vi "SetMotorOutFast.vi"(6 "Period (ms)":i32, 8 "error in (no error)":errorcluster, 9 "Sync Group / Parameter Slot":u8, 10 "Output":dbl, 11 "MotorControlDevRef":T1={"DeviceStatus"={"status"=FALSE, "code"=0, "source"=""}, "Type"=enum."PWM", "PWM"={"Controller"=enum."Controller 1", "PWM Channel"=enum."Invalid", "DeadBand"={"Name"="", "maxPositivePwm"=0, "minPositivePwm"=0, "centerPwm"=0, "maxNegativePwm"=0, "minNegativePwm"=0, "angularRange"=0}}, "CAN"={"Device Number"=0, "Control Mode"=enum."Percent VBus", "Semaphore"=refnum, "Max Vout"=12.0, "TalonSRX Control Mode"=enum."Percent VBus"}, "Invert"=FALSE, "TransformRef"=refnum, "InvTransformRef"=refnum}) -> (0 "error out":errorcluster, 2 "Motor Output":dbl, 3 "MotorControlDevRefOut":T1={"DeviceStatus"={"status"=FALSE, "code"=0, "source"=""}, "Type"=enum."PWM", "PWM"={"Controller"=enum."Controller 1", "PWM Channel"=enum."Invalid", "DeadBand"={"Name"="", "maxPositivePwm"=0, "minPositivePwm"=0, "centerPwm"=0, "maxNegativePwm"=0, "minNegativePwm"=0, "angularRange"=0}}, "CAN"={"Device Number"=0, "Control Mode"=enum."Percent VBus", "Semaphore"=refnum, "Max Vout"=12.0, "TalonSRX Control Mode"=enum."Percent VBus"}, "Invert"=FALSE, "TransformRef"=refnum, "InvTransformRef"=refnum})   [LabVIEW 2014]
uses:
  <vilib>/Rock Robotics/WPI/MotorControl/WPI_MotorControlDeviceRef.ctl
  <vilib>/Rock Robotics/WPI/MotorControl/WPI_MotorControlType.ctl
  <vilib>/Rock Robotics/SystemInterfaces/Typedef/FPGA_TypedefDigitalModule.ctl
  <vilib>/Rock Robotics/SystemInterfaces/DIO/FPGA_DIOPWMChannel.ctl
  <vilib>/Rock Robotics/WPI/PWM/WPI_PWMDeadband.ctl
  <vilib>/Rock Robotics/WPI/CAN/Jaguar/SubVIs/WPI_CANJaguar_ControlMode.ctl
  <vilib>/Rock Robotics/WPI/CAN/TalonSRX/WPI_CANTalonSRX_APIControlMode.ctl
  <vilib>/Rock Robotics/WPI/PWM/WPI_PWMTransform_ConPane.ctl
  <vilib>/Rock Robotics/WPI/CAN/Jaguar/SubVIs/WPI_CAN_TokenMessageIDs.ctl
  <vilib>/Rock Robotics/WPI/CAN/TalonSRX/WPI_CANTalonSRX_GlobalOps.ctl
  <vilib>/Rock Robotics/WPI/MotorControl/WPI_MotorControlSafetyCheck.vi
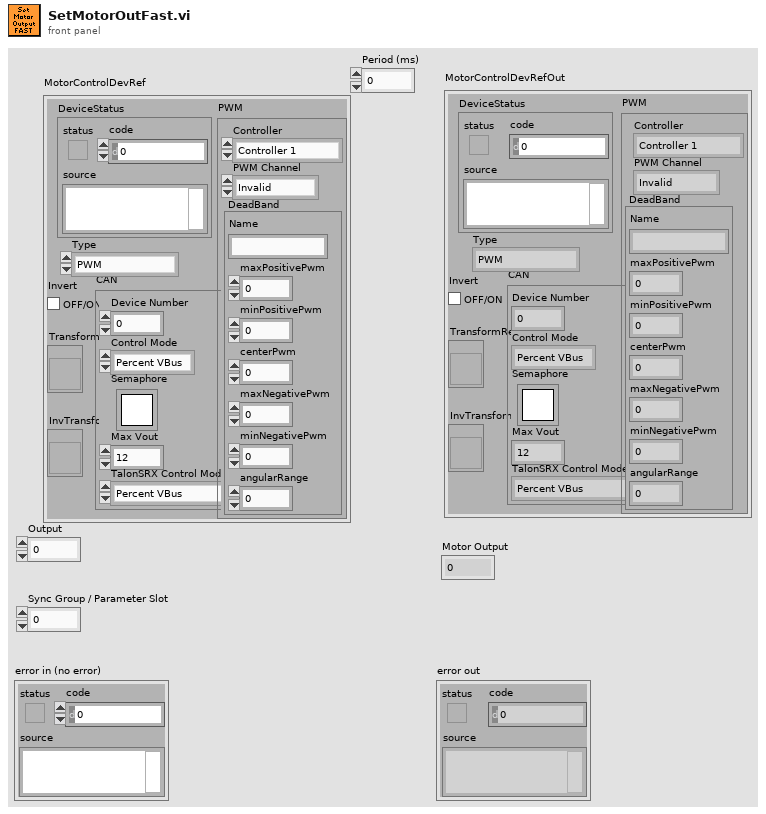
[diagram p1: front panel]
types:
  T1 = typedef "WPI_MotorControlDeviceRef.ctl" = cluster{"DeviceStatus":errorcluster, "Type":T2, "PWM":cluster{"Controller":T3, "PWM Channel":T4, "DeadBand":T5}, "CAN":cluster{"Device Number":u8, "Control Mode":T6, "Semaphore":T7, "Max Vout":dbl, "TalonSRX Control Mode":T8}, "Invert":bool, "TransformRef":T9, "InvTransformRef":T9}
  T2 = typedef "WPI_MotorControlType.ctl" = enum16{"PWM", "CAN", "CANTalonSRX"}
  T3 = typedef "FPGA_TypedefDigitalModule.ctl" = enum16{"Controller 1"}
  T4 = typedef "FPGA_DIOPWMChannel.ctl" = enum8{"PWM 0", "PWM 1", "PWM 2", "PWM 3", "PWM 4", "PWM 5", "PWM 6", "PWM 7", "PWM 8", "PWM 9", "PWM MXP 0", "PWM MXP 1", "PWM MXP 2", "PWM MXP 3", "PWM MXP 4", "PWM MXP 5", "PWM MXP 6", "PWM MXP 7", "PWM MXP 8", "PWM MXP 9", "Invalid"}
  T5 = typedef "WPI_PWMDeadband.ctl" = cluster{"Name":string, "maxPositivePwm":i32, "minPositivePwm":i32, "centerPwm":i32, "maxNegativePwm":i32, "minNegativePwm":i32, "angularRange":u16}
  T6 = typedef "WPI_CANJaguar_ControlMode.ctl" = enum8{"Percent VBus", "Current", "Speed", "Position", "Voltage"}
  T7 = typedef "Semaphore RefNum" = refnum<k1>
  T8 = typedef "WPI_CANTalonSRX_APIControlMode.ctl" = enum8{"Percent VBus", "Speed", "Position", "Slave", "Unchanged / Invalid"}
  T9 = typedef "WPI_PWMTransform_ConPane.ctl" = refnum<vi>
  T10 = enum16{"big-endian, network order", "native, host order", "little-endian"}
  T11 = typedef "WPI_CANTalonSRX_GlobalOps.ctl" = enum16{"Read For Send", "Write After Receive General", "Write After Receive Feedback", "Write After Receive Encoder", "Write After Receive Ain", "Write Error", "Get All", "Set Output", "Set Mode", "Set Master ID", "Set Brake Mode", "Set Reverse Feedback Sensor", "Set Reverse Closed Loop Output", "Set Override Limits", "Set Forward Limit Enabled", "Set Reverse Limit Enabled", "Set Feedback Select", "Set Profile Select", "Set Throttle Ramp Rate", "Disable"}
  T12 = typedef "WPI_PWMDeviceRef.ctl" = cluster{"DeviceStatus":errorcluster, "Controller":T3, "PWM Channel":T4}
  T13 = typedef "WPI_CAN_TokenMessageIDs.ctl" = u32
  T14 = typedef "WPI_CANTalonSRX_GlobalStatus.ctl" = cluster{"Applied Throttle":dbl, "Module Enabled":bool, "CAN Error":errorcluster, "Closed Loop Error":dbl, "Forward Limit Switch Closed":bool, "Reverse Limit Switch Closed":bool, "Sensor Position":dbl, "Sensor Velocity":dbl, "Current":dbl, "Sticky Fault - Over Temp":bool, "Sticky Fault - Under Voltage":bool, "Sticky Fault - Forward Limit":bool, "Sticky Fault - Reverse Limit":bool, "Sticky Fault - Forward Soft Limit":bool, "Sticky Fault - Reverse Soft Limit":bool, "Brake is Enabled":bool, "Encoder Position":dbl, "Encoder Velocity":dbl, "Encoder Index Count":dbl, "Encoder A Pin State":bool, "Encoder B Pin State":bool, "Encoder Index Pin State":bool, "Analog In":dbl, "Analog In Velocity":dbl, "Temperature (C)":dbl, "Battery Voltage":dbl}
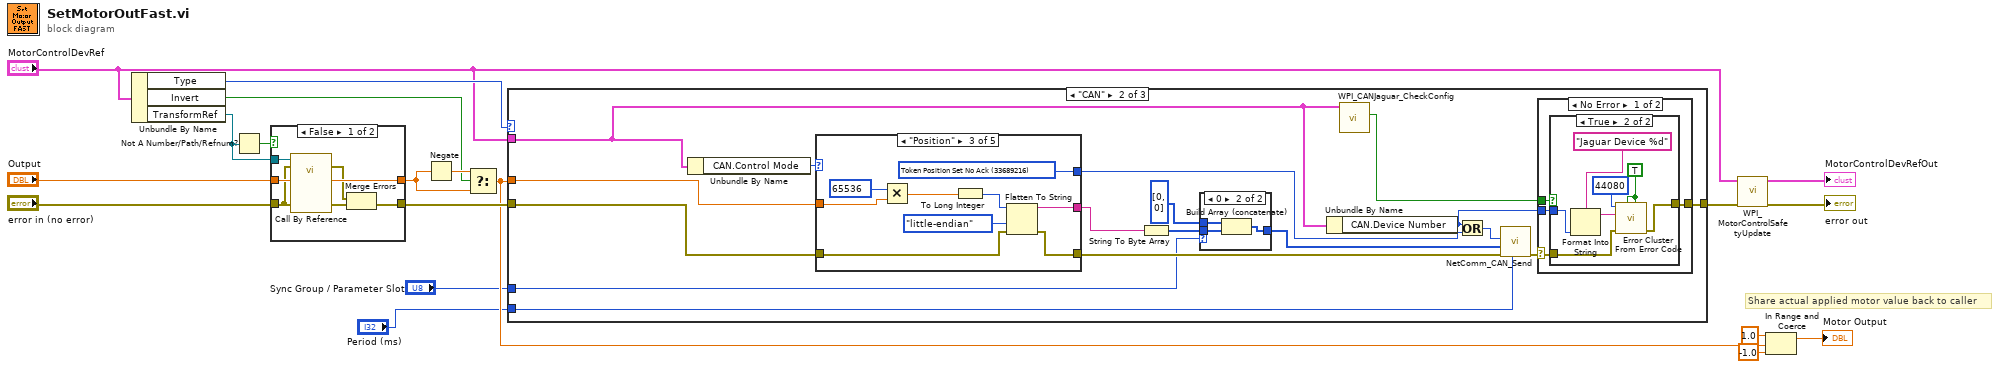
[diagram p0: block diagram]
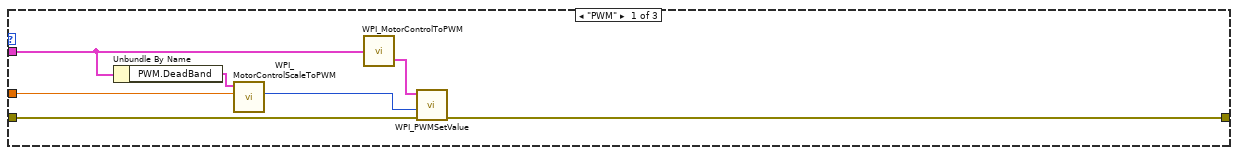
[diagram p3: hidden frame]
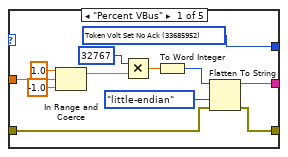
[diagram p6: hidden frame]
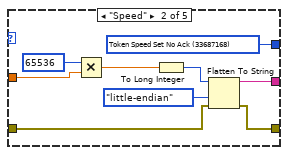
[diagram p7: hidden frame]
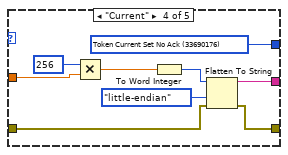
[diagram p8: hidden frame]
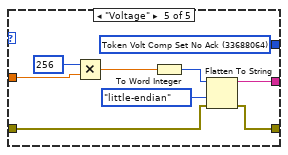
[diagram p9: hidden frame]
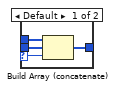
[diagram p10: hidden frame]
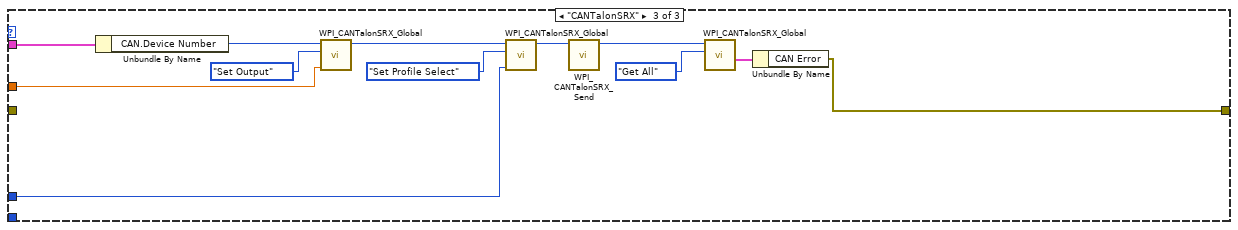
[diagram p11: hidden frame]
diagram:
  # "Share actual applied motor value back to caller"
  n1 = Unbundle By Name("MotorControlDevRef") -> ("Type"=w10:T2, "Invert"=w11:bool, "TransformRef"=w14:T9)
  n2 = Not A Number/Path/Refnum?(number/path/refnum=w14) -> (NaN/Path/Refnum?=w8:bool)
  n3 = case shown="False" w8 {
    tunnel: "Output" -> [w26 w28]
    tunnel: [w22 w27] -> w15
    tunnel: w14 -> [w25 _]
    tunnel: [w24 w28] -> w13
    tunnel: "error in (no error)" -> [w23 w27]
    frame False {
      n4 = call-by-ref "?"(reference=w25, error in=w23, 8:"error in (no error)"=w23, "Value in (1,-1)"=w26) -> (error out=w20:errorcluster, 0:"error out"=w21:errorcluster, "Value out (1,-1)"=w24:dbl)  [unwired: 8 in, 1 out]
      n5 = Merge Errors(w20, w21) -> (w22:errorcluster)
    }
    frame True {
    }
  }
  n6 = Negate(x=w13) -> (-x=w12:dbl)
  n7 = Select(t=w12, s=w11, f=w13) -> (s? t:f=w4:dbl)
  n8 = case shown="\"CAN\"" w10 {
    tunnel: w15 -> [w35 w47 _]
    tunnel: w4 -> [w33 w46 w129]
    tunnel: [w32 w39 w125] -> w9
    tunnel: "MotorControlDevRef" -> [w30 w42 w132]
    tunnel: "Sync Group / Parameter Slot" -> [_ w37 w121]
    tunnel: "Period (ms)" -> [_ w36 _]
    frame "PWM" {
      n9 = Unbundle By Name(w30) -> ("PWM.DeadBand"=w31:T5)
      n10 = call <vilib>:"WPI_MotorControlScaleToPWM.vi"("Output (1,-1)"=w33, "DeadBand Info"=w31) -> ("Raw PWM Value"=w34:u16)  [unwired: 9 out]
      n11 = call <vilib>:"WPI_MotorControlToPWM.vi"("MotorControlDeviceRef"=w30) -> ("PWMDeviceRef"=w29:T12)  [unwired: 1 out]
      n12 = call <vilib>:"WPI_PWMSetValue.vi"("error in (no error)"=w35, "Value"=w34, "PWMDeviceRef"=w29) -> ("error out"=w32:errorcluster)  [unwired: 1 in, 7 out]
    }
    frame "CAN" {
      n13 = Unbundle By Name(w42) -> ("CAN.Control Mode"=w44:T6)
      n14 = case shown="\"Position\"" w44 {
        tunnel: [w66 w78 w87 w96 w105] -> w52
        tunnel: w46 -> [w67 w80 w89 w99 w108]
        tunnel: w47 -> [w74 w84 w92 w103 w112]
        tunnel: [w73 w83 w91 w102 w111] -> w50
        tunnel: [w68 w82 w93 w101 w110] -> w45
        frame "Percent VBus" {
          w66 = T13 33685952 items=["Token Volt Enable"=33685760, "Token Volt Set"=33685824, "Token Volt Set No Ack"=33685952, "Token Speed Enable"=33686976, "Token Speed Set"=33687040, "Token Speed Set No Ack"=33687168, "Token Volt Comp Enable"=33687872, "Token Volt Comp Set"=33687936, "Token Volt Comp Set No Ack"=33688064, "Token Position Enable"=33689024, "Token Position Set"=33689088, "Token Position Set No Ack"=33689216, "Token Current Enable"=33689984, "Token Current Set"=33690048, "Token Current Set No Ack"=33690176] ("CAN Token Message IDs")
          n15 = In Range and Coerce(upper limit=1.0, x=w67, lower limit=-1.0) -> (coerced(x)=w72:dbl)  [unwired: 1 out]
          n16 = Multiply(x=i16 32767, y=w72) -> (x*y=w70:dbl)
          n17 = To Word Integer(number=w70) -> (16bit integer=w69:i16)
          n18 = Flatten To String(anything=w69, byte order (0:big-endian, network order)=T10."little-endian", error in (no error)=w74) -> (data string=w68:string, error out=w73:errorcluster)  [unwired: 2 out]
        }
        frame "Speed" {
          w78 = T13 33687168 items=["Token Volt Enable"=33685760, "Token Volt Set"=33685824, "Token Volt Set No Ack"=33685952, "Token Speed Enable"=33686976, "Token Speed Set"=33687040, "Token Speed Set No Ack"=33687168, "Token Volt Comp Enable"=33687872, "Token Volt Comp Set"=33687936, "Token Volt Comp Set No Ack"=33688064, "Token Position Enable"=33689024, "Token Position Set"=33689088, "Token Position Set No Ack"=33689216, "Token Current Enable"=33689984, "Token Current Set"=33690048, "Token Current Set No Ack"=33690176] ("CAN Token Message IDs")
          n19 = Multiply(x=u32 65536, y=w80) -> (x*y=w79:dbl)
          n20 = To Long Integer(number=w79) -> (32bit integer=w86:i32)
          n21 = Flatten To String(anything=w86, byte order (0:big-endian, network order)=T10."little-endian", error in (no error)=w84) -> (data string=w82:string, error out=w83:errorcluster)  [unwired: 2 out]
        }
        frame "Position" {
          w87 = T13 33689216 items=["Token Volt Enable"=33685760, "Token Volt Set"=33685824, "Token Volt Set No Ack"=33685952, "Token Speed Enable"=33686976, "Token Speed Set"=33687040, "Token Speed Set No Ack"=33687168, "Token Volt Comp Enable"=33687872, "Token Volt Comp Set"=33687936, "Token Volt Comp Set No Ack"=33688064, "Token Position Enable"=33689024, "Token Position Set"=33689088, "Token Position Set No Ack"=33689216, "Token Current Enable"=33689984, "Token Current Set"=33690048, "Token Current Set No Ack"=33690176] ("CAN Token Message IDs")
          n22 = Multiply(x=u32 65536, y=w89) -> (x*y=w88:dbl)
          n23 = To Long Integer(number=w88) -> (32bit integer=w94:i32)
          n24 = Flatten To String(anything=w94, byte order (0:big-endian, network order)=T10."little-endian", error in (no error)=w92) -> (data string=w93:string, error out=w91:errorcluster)  [unwired: 2 out]
        }
        frame "Current" {
          w96 = T13 33690176 items=["Token Volt Enable"=33685760, "Token Volt Set"=33685824, "Token Volt Set No Ack"=33685952, "Token Speed Enable"=33686976, "Token Speed Set"=33687040, "Token Speed Set No Ack"=33687168, "Token Volt Comp Enable"=33687872, "Token Volt Comp Set"=33687936, "Token Volt Comp Set No Ack"=33688064, "Token Position Enable"=33689024, "Token Position Set"=33689088, "Token Position Set No Ack"=33689216, "Token Current Enable"=33689984, "Token Current Set"=33690048, "Token Current Set No Ack"=33690176] ("CAN Token Message IDs")
          n25 = Multiply(x=u32 256, y=w99) -> (x*y=w98:dbl)
          n26 = To Word Integer(number=w98) -> (16bit integer=w100:i16)
          n27 = Flatten To String(anything=w100, byte order (0:big-endian, network order)=T10."little-endian", error in (no error)=w103) -> (data string=w101:string, error out=w102:errorcluster)  [unwired: 2 out]
        }
        frame "Voltage" {
          w105 = T13 33688064 items=["Token Volt Enable"=33685760, "Token Volt Set"=33685824, "Token Volt Set No Ack"=33685952, "Token Speed Enable"=33686976, "Token Speed Set"=33687040, "Token Speed Set No Ack"=33687168, "Token Volt Comp Enable"=33687872, "Token Volt Comp Set"=33687936, "Token Volt Comp Set No Ack"=33688064, "Token Position Enable"=33689024, "Token Position Set"=33689088, "Token Position Set No Ack"=33689216, "Token Current Enable"=33689984, "Token Current Set"=33690048, "Token Current Set No Ack"=33690176] ("CAN Token Message IDs")
          n28 = Multiply(x=u32 256, y=w108) -> (x*y=w107:dbl)
          n29 = To Word Integer(number=w107) -> (16bit integer=w109:i16)
          n30 = Flatten To String(anything=w109, byte order (0:big-endian, network order)=T10."little-endian", error in (no error)=w112) -> (data string=w110:string, error out=w111:errorcluster)  [unwired: 2 out]
        }
      }
      n31 = String To Byte Array(string=w45) -> (unsigned byte array=w48:u8[])
      n32 = case shown="0" w37 {
        selector: w37 -> [w114 _]
        tunnel: [w117 w120] -> w51
        tunnel: u8[] [0, 0] ("data") -> [w116 w119]
        tunnel: w48 -> [w115 w118]
        frame Default {
          n33 = Build Array (concatenate)(w116, w115, w114) -> (w117:u8[])
        }
        frame 0 {
          n34 = Build Array (concatenate)(w119, w118) -> (w120:u8[])
        }
      }
      n35 = Unbundle By Name(w42) -> ("CAN.Device Number"=w38:u8)
      n36 = call <vilib>:"WPI_CANJaguar_CheckConfig.vi"("CAN Jaguar Ref"=w42) -> ("Warning"=w40:bool)  [unwired: 10 in]
      n37 = Or(x=w38, y=w52) -> (x .or. y?=w43:T13)
      n38 = call <vilib>:"NetComm_CAN_Send.vi"("Period (ms)"=w36, "error in (no error)"=w50, "Data"=w51, "Message ID"=w43) -> ("error out"=w41:errorcluster)  [unwired: 7 out]
      n39 = case shown="No Error" w41 {
        selector: w41 -> [w56 w65]
        tunnel: w40 -> [w53 _]
        tunnel: [w55 w65] -> w39
        tunnel: w38 -> [w54 _]
        frame No Error {
          n40 = case shown="True" w53 {
            tunnel: w56 -> [w57 w62]
            tunnel: [w57 w61] -> w55
            tunnel: w54 -> [_ w58]
            frame False {
            }
            frame True {
              w63 = TRUE ("is warning? (False)")
              n41 = Format Into String(format string="Jaguar Device %d", w58) -> (resulting string=w60:string)  [unwired: 2 in, 1 out]
              n42 = call <vilib>:"Error Cluster From Error Code.vi"("is warning? (False)"=w63, "show call chain? (False)"=w63, "error in (no error)"=w62, "error message (\"\")"=w60, "error code (0)"=44080) -> ("error out"=w61:errorcluster)  [unwired: 4 in]
            }
          }
        }
        frame Error {
        }
      }
    }
    frame "CANTalonSRX" {
      n43 = Unbundle By Name(w132) -> ("CAN.Device Number"=w131:u8)
      n44 = call <vilib>:"WPI_CANTalonSRX_Global.vi"("Set Number"=w129, "Operation"=WPI_CANTalonSRX_GlobalOps."Set Output", "Device ID (0)"=w131) -> ("Device ID Out"=w123:u8)  [unwired: 6 in, 2 out]
      n45 = call <vilib>:"WPI_CANTalonSRX_Global.vi"("Set Number"=w121, "Operation"=WPI_CANTalonSRX_GlobalOps."Set Profile Select", "Device ID (0)"=w123) -> ("Device ID Out"=w122:u8)  [unwired: 6 in, 2 out]
      n46 = call <vilib>:"WPI_CANTalonSRX_Send.vi"("Device ID (0)"=w122) -> ("Device ID Out"=w128:u8)  [unwired: 10 in]
      n47 = call <vilib>:"WPI_CANTalonSRX_Global.vi"("Operation"=WPI_CANTalonSRX_GlobalOps."Get All", "Device ID (0)"=w128) -> ("Get All"=w126:T14)  [unwired: 7 in, 2 out]
      n48 = Unbundle By Name(w126) -> ("CAN Error"=w125:errorcluster)
    }
  }
  n49 = call <vilib>:"WPI_MotorControlSafetyUpdate.vi"("error in (no error)"=w9, "MotorControlDevRef"="MotorControlDevRef") -> ("error out"=→"error out":errorcluster, "MotorControlDevRef"=→"MotorControlDevRefOut":T1)  [unwired: 8 out]
  n50 = In Range and Coerce(upper limit=1.0, x=w4, lower limit=-1.0) -> (coerced(x)=→"Motor Output":dbl)  [unwired: 1 out]
